vi "Destroy.vi"(0 "reference in":refnum<class "MyPropertyClass_LV2010.lvclass">, 5 "error in (no error)":errorcluster) -> (14 "reference out":refnum<class "MyPropertyClass_LV2010.lvclass">, 19 "error out":errorcluster)   [LabVIEW 2017, in "MyPropertyClass_LV2010.lvclass"]
doc: "Destructor."
uses:
  MyPropertyClass_LV2010.lvclass
  vi.lib/addons/_AddQ/G#Object/G#Object.lvclass
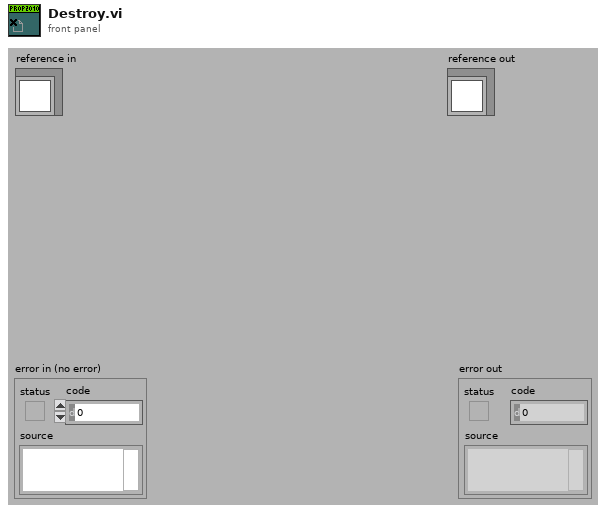
[diagram p1: front panel]
types:
  T1 = typedef "MyPropertyClass_LV2010.lvclass/ObjectAttributes.ctl" = cluster{"MyAttribute":dbl, "Name":string}
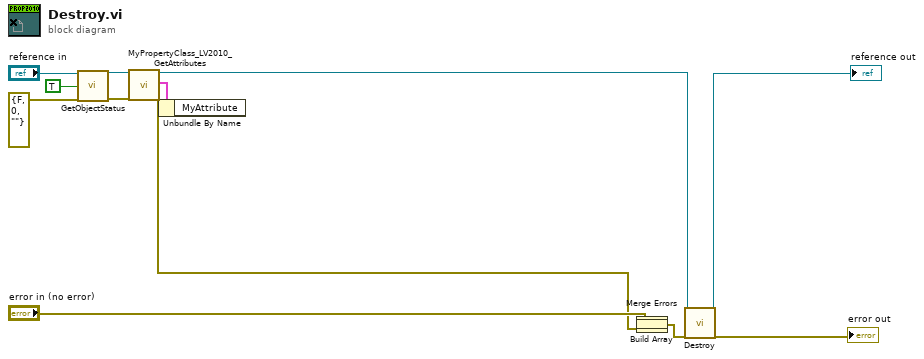
[diagram p0: block diagram]
diagram:
  n1 = call-dynamic "GetObjectStatus.vi"("reference in"="reference in", "simple info (F)"=TRUE ("simple info"), "error in (no error)"=errorcluster {"status"=FALSE, "code"=0, "source"=""}) -> ("reference out"=w6:refnum<class "MyPropertyClass_LV2010.lvclass">, "error out"=w7:errorcluster)  [unwired: 5 in, 10 out]
  n2 = call "MyPropertyClass_LV2010_GetAttributes.vi"("reference in"=w6, "error in (no error)"=w7) -> ("reference out"=w5:refnum<class "MyPropertyClass_LV2010.lvclass">, "attributes"=w4:T1, "error out"=w8:errorcluster)  [unwired: 14 in, 1 out]
  n3 = Unbundle By Name(w4) -> ()  [unwired: 1 out]
  n4 = Build Array("error in (no error)", w8) -> (w1:errorcluster[])
  n5 = Merge Errors(w1) -> (w12:errorcluster)
  n6 = call-parent "Destroy.vi"("reference in"=w5, "error in (no error)"=w12) -> ("reference out"=→"reference out":refnum<class "MyPropertyClass_LV2010.lvclass">, "error out"=→"error out":errorcluster)  [unwired: 16 in]
